vi "Draw.vi"(8 "error in (no error)":errorcluster, 11 "Circle in":refnum<class "PacMan.lvclass">) -> (0 "error out":errorcluster, 3 "Circle out":refnum<class "PacMan.lvclass">)   [LabVIEW 2016, in "PacManClasses.lvlib" / "PacMan.lvclass"]
uses:
  PacMan.lvclass
  C:/Users/lucamach/Documents/SE/Learning OOP/PacMan/PacMan Classes/Geometric Figure/UI Object.lvclass
  Geometric Figure/UI Object.lvclass/UI Object.ctl
  Geometric Figure/Read Center (px).vi
  Geometric Figure/Read Color (RGB).vi
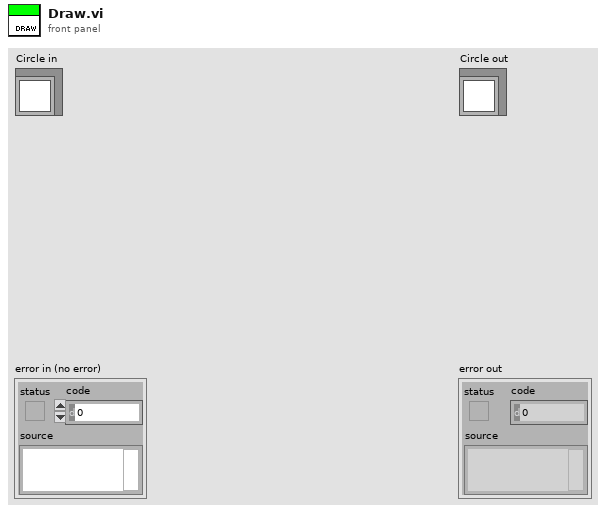
[diagram p1: front panel]
types:
  T1 = typedef "PacManClasses.lvlib/Picture.ctl" = picture
  T2 = typedef "PacManClasses.lvlib/Size - Bounding Rect.ctl" = cluster{"Width":u16, "Height":u16}
  T3 = typedef "PacManClasses.lvlib/Point.ctl" = cluster{"x":u16, "y":u16}
  T4 = typedef "PacManClasses.lvlib/Color.ctl" = cluster{"Red":u8, "Green":u8, "Blue":u8}
  T5 = typedef "PacManClasses.lvlib/Pen.ctl" = cluster{"Width":u16, "Style":enum32{"Solid", "Dash", "Dot", "DashDot", "DashDotDot"}}
  T6 = typedef "PacManClasses.lvlib/PacMan Arc.ctl" = cluster{"Start Angle (°)":i16, "Arc Size (°)":i16}
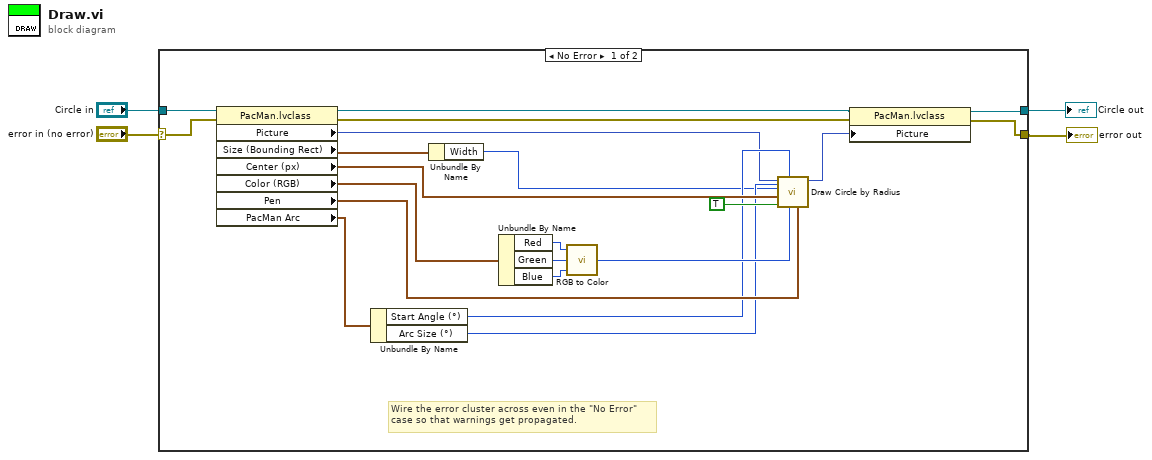
[diagram p0: block diagram]
diagram:
  n1 = case shown="No Error" "error in (no error)" {
    selector: "error in (no error)" -> [w16 w27]
    tunnel: [w6 w27] -> w1
    tunnel: [w5 w26] -> w3
    tunnel: "Circle in" -> [w20 w26]
    frame No Error {
      # "Wire the error cluster across even in the \"No Error\"\ncase so that warnings get propagated."
      n2 = property class="PacMan.lvclass"(reference=w20, error in=w16) -> (reference out=w9:refnum<class "PacMan.lvclass">, error out=w7:errorcluster, "Picture"=w12:T1, "Size (Bounding Rect)"=w11:T2, "Center (px)"=w19:T3, "Color (RGB)"=w18:T4, "Pen"=w17:T5, "PacMan Arc"=w15:T6)
      n3 = Unbundle By Name(w15) -> ("Start Angle (°)"=w14:i16, "Arc Size (°)"=w13:i16)
      n4 = Unbundle By Name(w11) -> ("Width"=w10:u16)
      n5 = Unbundle By Name(w18) -> ("Red"=w24:u8, "Green"=w23:u8, "Blue"=w22:u8)
      n6 = call <vilib>:"RGB to Color.vi"("B"=w22, "G"=w23, "R"=w24) -> ("Color"=w25:u32)
      n7 = call <vilib>:"Draw Circle by Radius.vi"("pen"=w17, "arc size(360)"=w13, "color(black)"=w25, "start angle(0)"=w14, "fill?(F)"=TRUE, "pixel center"=w19, "radius"=w10, "picture"=w12) -> ("new picture"=w8:picture)  [unwired: 3 in]
      n8 = property class="PacMan.lvclass"(reference=w9, error in=w7, "Picture"=w8) -> (reference out=w5:refnum<class "PacMan.lvclass">, error out=w6:errorcluster)
    }
    frame Error {
    }
  }
  "error out" <- w1
  "Circle out" <- w3
